vi "Gantner_DecodeModules.vi"(8 "error in":errorcluster caption="Fehler (Eingang - kein Fehler)", 9 "Array":i32[](array[numeric]), 10 "ItemsCount":i32, 11 "Stricture ID":i32) -> (0 "error out":errorcluster caption="Fehler (Ausgang)", 3 "ModuleArray":T1[](array[typedef]))   [LabVIEW 2016]
uses:
  Gantner-Instruments ISMBUS32/ISMBUS_Module.ctl
  Gantner-Instruments ISMBUS32/ISMBUS_Channel.ctl
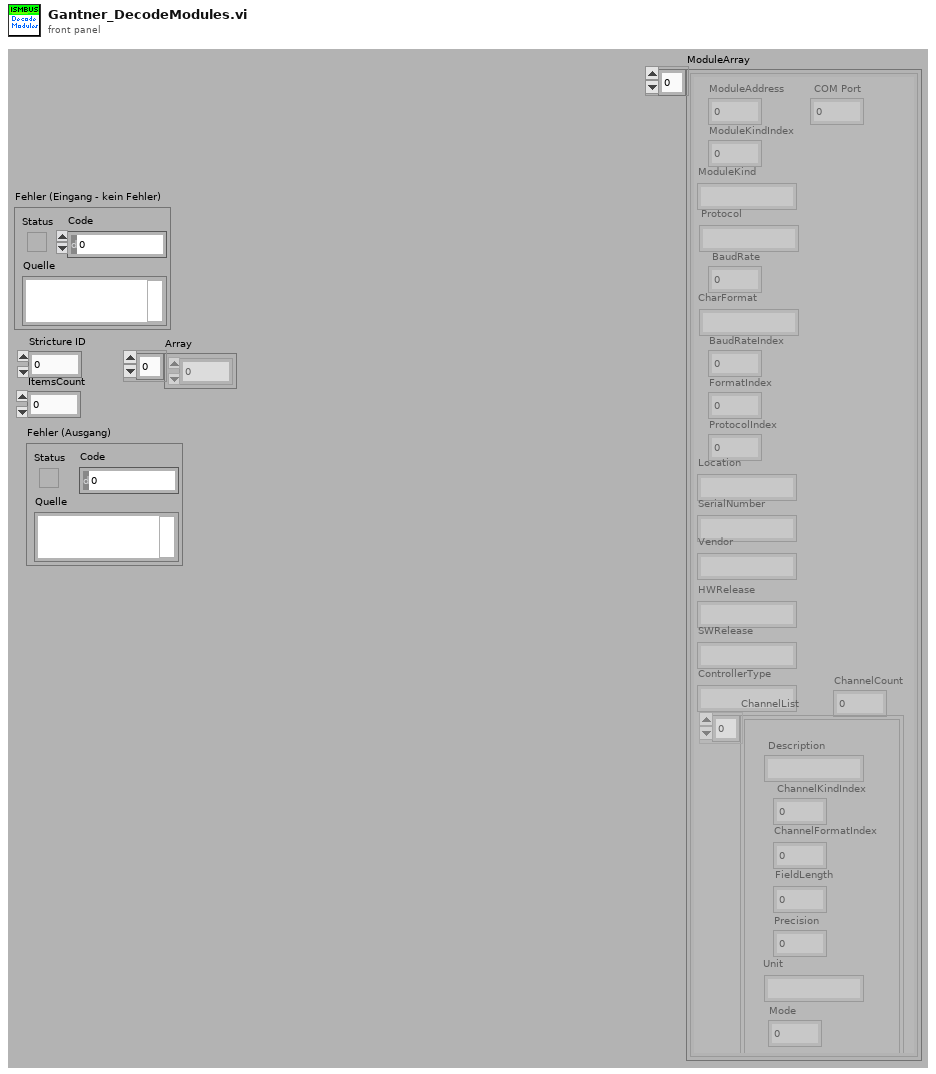
[diagram p1: front panel]
types:
  T1 = typedef "ISMBUS_Module.ctl" = cluster{"ModuleAddress":i32, "ModuleKindIndex":i32, "ModuleKind":string, " Protocol":string, " BaudRate":i32, "CharFormat":string, "BaudRateIndex":i32, "FormatIndex":i32, "ProtocolIndex":i32, "Location":string, "SerialNumber":string, "Vendor":string, "HWRelease":string, "SWRelease":string, "ControllerType":string, "ChannelList":T2[], "ChannelCount":i32, " COM Port":i32}
  T2 = typedef "ISMBUS_Channel.ctl" = cluster{" Description":string, " ChannelKindIndex":i32, "ChannelFormatIndex":i32, " FieldLength":i32, "Precision":i32, "Unit":string, "Mode":i32}
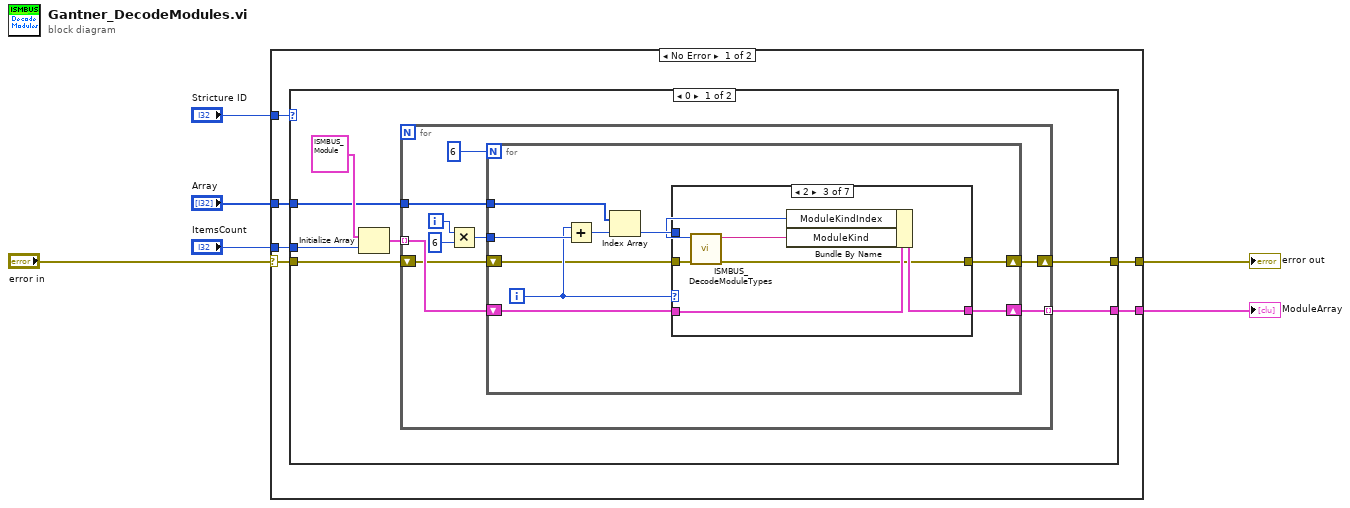
[diagram p0: block diagram]
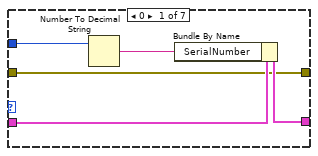
[diagram p2: hidden frame]
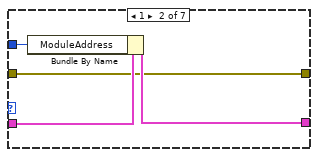
[diagram p3: hidden frame]
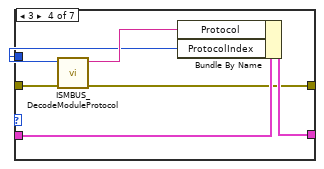
[diagram p4: hidden frame]
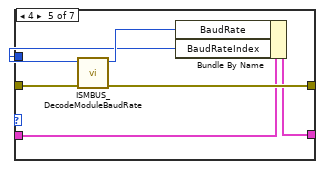
[diagram p5: hidden frame]
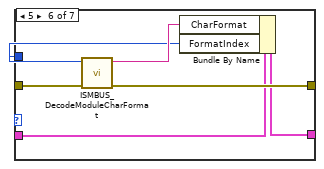
[diagram p6: hidden frame]
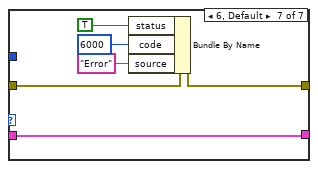
[diagram p7: hidden frame]
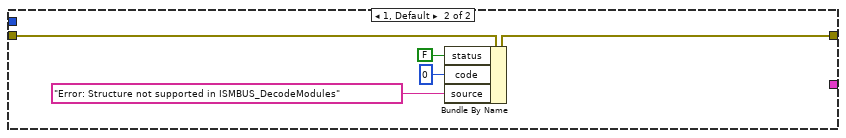
[diagram p8: hidden frame]
diagram:
  n1 = case shown="No Error" "error in" {
    selector: "error in" -> [w11 w82]
    tunnel: "Stricture ID" -> [w12 _]
    tunnel: "ItemsCount" -> [w9 _]
    tunnel: "Array" -> [w10 _]
    tunnel: [w8 _] -> w1
    tunnel: [w7 w82] -> w2
    frame No Error {
      n2 = case shown="0" w12 {
        tunnel: w11 -> [w14 w80]
        tunnel: w10 -> [w16 _]
        tunnel: w9 -> [w18 _]
        tunnel: [w15 _] -> w8
        tunnel: [w13 w81] -> w7
        frame 0 {
          n3 = Initialize Array(T1 {"ModuleAddress"=0, "ModuleKindIndex"=0, "ModuleKind"="", " Protocol"="", " BaudRate"=0, "CharFormat"="", "BaudRateIndex"=0, "FormatIndex"=0, "ProtocolIndex"=0, "Location"="", "SerialNumber"="", "Vendor"="", "HWRelease"="", "SWRelease"="", "ControllerType"="", "ChannelList"=[], "ChannelCount"=0, " COM Port"=0} ("Module"), w18) -> (w17:T1[])
          n4 = for {
            tunnel: w17 -> [w22] mode=indexing
            tunnel: w16 -> [w24]
            tunnel: [w23] -> w15 mode=indexing
            shift-right: [w20] -> w13
            shift-left: w14 -> [w21]
            i -> [w28]
            n5 = Multiply(x=w28, y=6) -> (x*y=w26:i32)
            n6 = for {
              N: 6 -> [_]
              tunnel: w26 -> [w37]
              tunnel: w24 -> [w36]
              shift-right: [w31] -> w23
              shift-left: w22 -> [w32]
              shift-right: [w29] -> w20
              shift-left: w21 -> [w30]
              i -> [w34]
              n7 = Add(x=w34, y=w37) -> (x+y=w35:i32)
              n8 = Index Array(array=w36, index=w35) -> (element=w33:i32)
              n9 = case shown="2" w34 {
                tunnel: w33 -> [w39 w44 w50 w53 w59 w65 _]
                tunnel: w32 -> [w41 w46 w52 w57 w61 w67 w76]
                tunnel: [w42 w45 w51 w58 w62 w68 w76] -> w31
                tunnel: w30 -> [w40 w43 w48 w55 w64 w70 w74]
                tunnel: [w40 w43 w47 w54 w63 w69 w75] -> w29
                frame 0 {
                  n10 = Number To Decimal String(number=w39) -> (decimal integer string=w38:string)  [unwired: 1 in]
                  n11 = Bundle By Name(cluster=w41, "SerialNumber"=w38) -> (w42:T1)
                }
                frame 1 {
                  n12 = Bundle By Name(cluster=w46, "ModuleAddress"=w44) -> (w45:T1)
                }
                frame 2 {
                  n13 = call "ISMBUS_DecodeModuleTypes.vi"("Fehler (Eingang - kein Fehler)"=w48, "ModuleKindIndex"=w50) -> ("error (Ausgang)"=w47:errorcluster, "ModulType String"=w49:string)  [unwired: 8 in]
                  n14 = Bundle By Name(cluster=w52, "ModuleKindIndex"=w50, "ModuleKind"=w49) -> (w51:T1)
                }
                frame 3 {
                  n15 = call "ISMBUS_DecodeModuleProtocol.vi"("Fehler (Eingang - kein Fehler)"=w55, "ModuleProtocolIndex"=w53) -> ("error (Ausgang)"=w54:errorcluster, "ModuleProtocolString"=w56:string)  [unwired: 8 in]
                  n16 = Bundle By Name(cluster=w57, "Protocol"=w56, "ProtocolIndex"=w53) -> (w58:T1)
                }
                frame 4 {
                  n17 = call "ISMBUS_DecodeModuleBaudRate.vi"("Fehler (Eingang - kein Fehler)"=w64, "ModuleBaudRate in"=w59) -> ("error (Ausgang)"=w63:errorcluster, "ModuleBaudRate in 2"=w60:i32)  [unwired: 8 in]
                  n18 = Bundle By Name(cluster=w61, "BaudRate"=w60, "BaudRateIndex"=w59) -> (w62:T1)
                }
                frame 5 {
                  n19 = call "ISMBUS_DecodeModuleCharFormat.vi"("Fehler (Eingang - kein Fehler)"=w70, "ModuleCharFormatIndex"=w65) -> ("error (Ausgang)"=w69:errorcluster, "ModuleCharFormatString"=w66:string)  [unwired: 8 in]
                  n20 = Bundle By Name(cluster=w67, "CharFormat"=w66, "FormatIndex"=w65) -> (w68:T1)
                }
                frame 6, Default {
                  n21 = Bundle By Name(cluster=w74, "status"=TRUE, "code"=6000, "source"="Error") -> (w75:errorcluster)
                }
              }
            }
          }
        }
        frame 1, Default {
          n22 = Bundle By Name(cluster=w80, "status"=FALSE, "code"=0, "source"="Error: Structure not supported in ISMBUS_DecodeModules") -> (w81:errorcluster)
        }
      }
    }
    frame Error {
    }
  }
  "ModuleArray" <- w1
  "error out" <- w2
